vi "Move Inc.vi"(6 "Axis":string, 8 "error in (no error)":errorcluster, 9 "Speed":dbl format="%#_13g", 10 "Distance":dbl format="%#_13g", 11 "Gantry In":refnum<k24>) -> (0 "error out":errorcluster, 3 "Gantry Out":refnum<k24>)   [LabVIEW 2019, in "A3200.lvclass"]
uses:
  A3200.lvclass
  C:/Program Files (x86)/Aerotech/A3200/LabVIEW/2010/Bin/Aerotech.A3200.dll
  Program Files (x86)/Aerotech/A3200/LabVIEW/2010/Bin/Aerotech.A3200.dll
  Drivers/Aerotech A3200/Aerotech VIs.lvlib
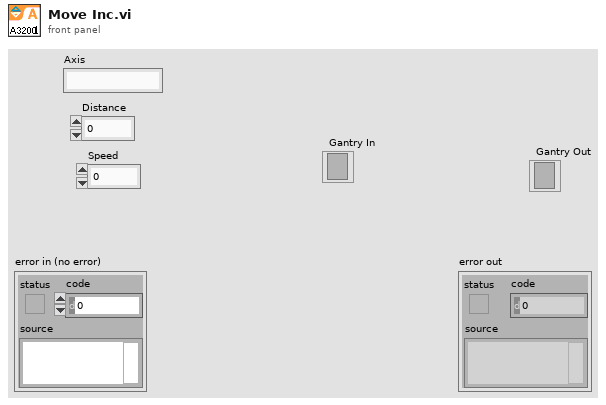
[diagram p1: front panel]
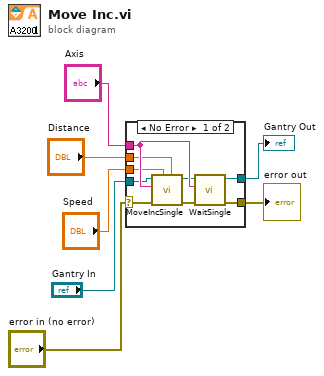
[diagram p0: block diagram]
diagram:
  n1 = case shown="No Error" "error in (no error)" {
    selector: "error in (no error)" -> [w10 w18]
    tunnel: [w8 w18] -> w6
    tunnel: "Axis" -> [w16 _]
    tunnel: "Speed" -> [w15 _]
    tunnel: "Distance" -> [w14 _]
    tunnel: "Gantry In" -> [w12 w17]
    tunnel: [w11 w17] -> w1
    frame No Error {
      n2 = call "MoveIncSingle.vi"("distance"=w14, "speed"=w15, "error in (no error)"=w10, "axis name"=w16, "controller in"=w12) -> ("error out"=w9:errorcluster, "controller out"=w13:refnum<k24>)  [unwired: 5 in]
      n3 = call "WaitSingle.vi"("error in (no error)"=w9, "axis name"=w16, "controller in"=w13) -> ("error out"=w8:errorcluster, "controller out"=w11:refnum<k24>)  [unwired: 6 in, 1 out]
    }
    frame Error {
    }
  }
  "error out" <- w6
  "Gantry Out" <- w1
